vi "switch_cont.vi"(7 "LabVIEW Web Service Request":refnum<class "Web Request.lvclass">) -> ()   [LabVIEW 2014]
uses:
  <vilib>/wsapi/Web Request.lvclass
  DataManager/StateStore/Controls/DataFunction.ctl
panel:
  # "Use the Web Service Request input terminal to call the VIs on the Web Services palette. Do not remove it from the connector pane unless you don't need access to the palette."
  # "Each additional control wired to the connector pane will be available as an input in the URL. To include an indicator in terminal-mode output (the default setting), it must also be wired to the connector pane."
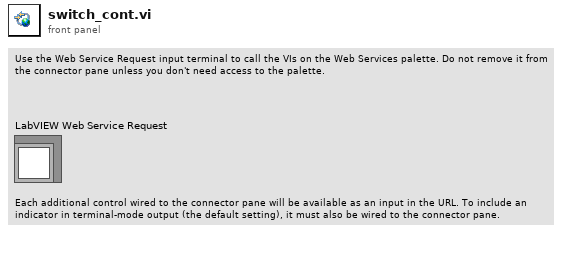
[diagram p1: front panel]
types:
  T1 = typedef "DataFunction.ctl" = enum16{"Initialise", "Release", "Get Data", "Set Data", "Preview Data"}
  T2 = typedef "CData Core Control.ctl" = cluster{"train_data_array":cluster{"uuid":string, "int":i32, "posit_array":cluster{"x":dbl, "y":dbl, "z":dbl}[]}[], "train_control_array":cluster{"uuid":string, "throttle":dbl, "brake":dbl, "horn":dbl, "wait":dbl, "name":string, "mode":string, "dest":string}[], "switch_data_array":cluster{"switch_posit":cluster{"x":dbl, "y":dbl, "z":dbl}, "manual":bool}[], "switch_control_array":cluster{"switch_posit":cluster{"x":dbl, "y":dbl, "z":dbl}, "switch":bool, "invert":bool, "wait":dbl}[]}
  T3 = cluster{"switch_posit":cluster{"x":dbl, "y":dbl, "z":dbl}, "switch":bool, "invert":bool, "wait":dbl}[]
  T4 = cluster{"switch_posit":cluster{"x":dbl, "y":dbl, "z":dbl}, "switch":bool, "invert":bool, "wait":dbl}
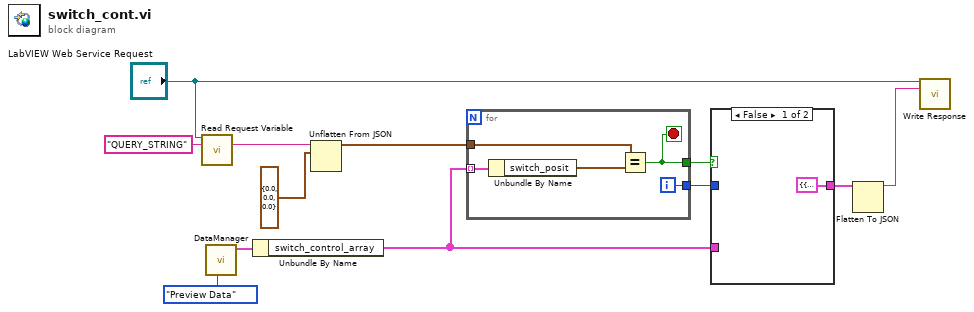
[diagram p0: block diagram]
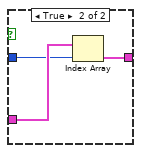
[diagram p2: hidden frame]
diagram:
  n1 = call <vilib>:"Read Request Variable.vi"("LabVIEW Web Service Request"="LabVIEW Web Service Request", "variable name"="QUERY_STRING") -> ("value"=w3:string)  [unwired: 11 in, 2 out]
  n2 = call "DataManager.vi"("DataFunction"=DataFunction."Preview Data") -> ("CData Out"=w11:T2)  [unwired: 9 in, 1 out]
  n3 = Unbundle By Name(w11) -> ("switch_control_array"=w8:T3)
  n4 = Unflatten From JSON(JSON string=w3, type and defaults=cluster{"x":dbl, "y":dbl, "z":dbl} {"x"=0.0, "y"=0.0, "z"=0.0} ("switch_posit")) -> (value=w1:cluster{"x":dbl, "y":dbl, "z":dbl})  [unwired: 5 in, 1 out]
  n5 = for {
    tunnel: w8 -> [w17] mode=indexing
    tunnel: w1 -> [w16]
    tunnel: [w15] -> w10
    tunnel: [w14] -> w9
    i -> [w14]
    stop <- w15 stop-if-true
    n6 = Unbundle By Name(w17) -> ("switch_posit"=w13:cluster{"x":dbl, "y":dbl, "z":dbl})
    n7 = Equal?(x=w16, y=w13) -> (x = y?=w15:bool)
  }
  n8 = case shown="False" w10 {
    tunnel: w9 -> [_ w20]
    tunnel: w8 -> [_ w21]
    tunnel: [T4 {"switch_posit"={"x"=0.0, "y"=0.0, "z"=0.0}, "switch"=FALSE, "invert"=FALSE, "wait"=0.0} ("switch_control") w19] -> w6
    frame False {
    }
    frame True {
      n9 = Index Array(array=w21, index=w20) -> (element=w19:T4)
    }
  }
  n10 = Flatten To JSON(anything=w6) -> (JSON string=w5:string)  [unwired: 2 in, 1 out]
  n11 = call <vilib>:"Write Response.vi"("LabVIEW Web Service Request"="LabVIEW Web Service Request", "response string"=w5) -> ()  [unwired: 12 in, 2 out]
